vi "Reset Buffer Size.vi"(4 "Error In":errorcluster, 6 "Instance Name":T1, 7 "New Buffer Size":i32) -> (0 "Error Out":errorcluster)   [LabVIEW 2015, in "Temperature Controller Data Buffer.lvlib"]
uses:
  Temperature Controller Data Buffer.lvlib
  _libraries/Startup Processes/_typedefs/Subpanel Names.ctl
  _libraries/Startup Processes/Startup Processes.lvlib
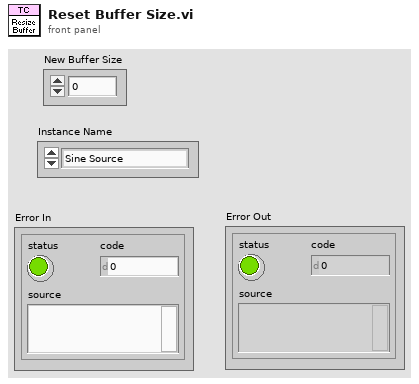
[diagram p1: front panel]
types:
  T1 = typedef "Startup Processes.lvlib/Subpanel Names.ctl" = enum16{"Sine Source", "Ramp Source", "Hen House TC", "Dog House TC", "Out House TC"}
  T2 = typedef "Temperature Controller Data Buffer.lvlib/buffer data typedef.ctl" = cluster{"TC Data":cluster{"Last value":dbl, "Error High Level":dbl, "Warning High Level":dbl, "Warning Low Level":dbl, "Error Low Level":dbl}[], "Counter":i32}
  T3 = cluster{"Last value":dbl, "Error High Level":dbl, "Warning High Level":dbl, "Warning Low Level":dbl, "Error Low Level":dbl}[]
  T4 = cluster{"Last value":dbl, "Error High Level":dbl, "Warning High Level":dbl, "Warning Low Level":dbl, "Error Low Level":dbl}
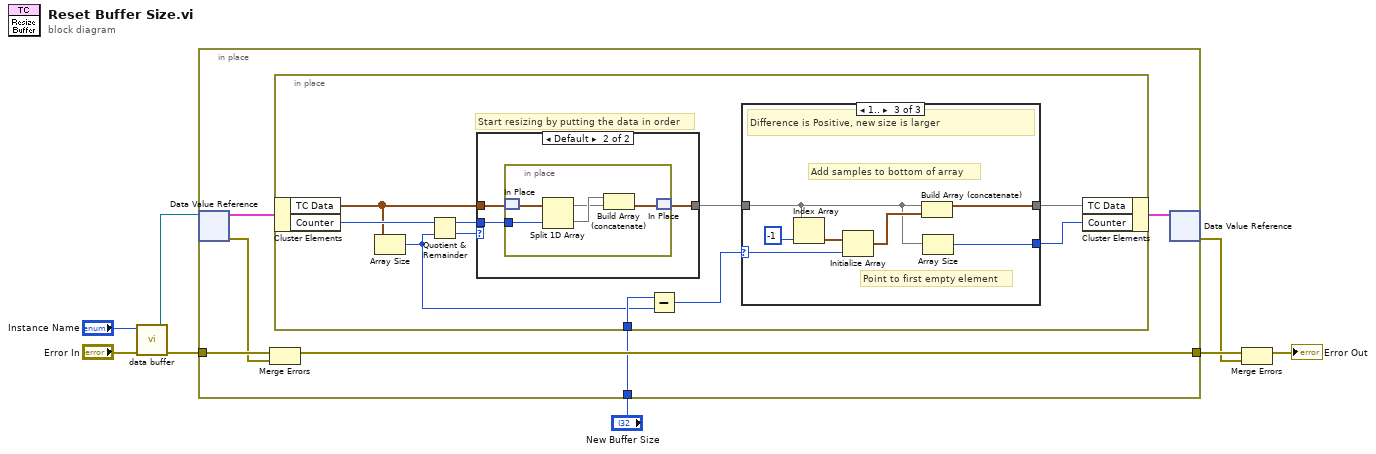
[diagram p0: block diagram]
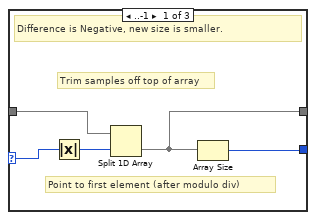
[diagram p2: hidden frame]
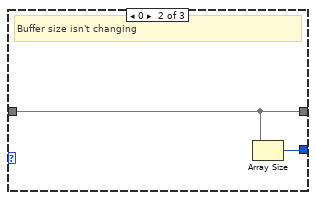
[diagram p3: hidden frame]
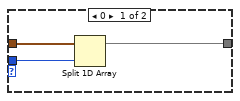
[diagram p4: hidden frame]
diagram:
  n1 = call "data buffer.vi"("Error In"="Error In", "Instance Name"="Instance Name") -> ("Error Out"=w6:errorcluster, "DVR"=w5:refnum<data-value>)  [unwired: 4 in]
  n2 = in-place {
    in-place-border: w6 -> [w14]
    in-place-border: [w13] -> w7
    in-place-border: "New Buffer Size" -> [w9]
    n3 = in-place-dvr #1(w5) -> (w11:T2, w12:errorcluster)
    n4 = Merge Errors(w14, w12) -> (w13:errorcluster)
    n5 = in-place {
      in-place-border: w9 -> [w16]
      # "Start resizing by putting the data in order"
      n6 = in-place-cluster #2(w11) -> ("TC Data"=w18:T3, "Counter"=w22:i32)
      n7 = Array Size(array=w18) -> (size(s)=w15:i32)
      n8 = Quotient & Remainder(x=w22, y=w15) -> (x-y*floor(x/y)=w23:i32, floor(x/y)=w24:i32)
      n9 = case shown="Default" w24 {
        tunnel: w18 -> [w41 w44]
        tunnel: [w39 w43] -> w21
        tunnel: w23 -> [w40 w42]
        frame 0 {
          n10 = Split 1D Array(array=w41, index=w40) -> (first subarray=w39:T3)  [unwired: 1 out]
        }
        frame Default {
          n11 = in-place {
            in-place-border: w42 -> [w49]
            n12 = in-place-match #3(w44) -> (w46:T3)
            n13 = Split 1D Array(array=w46, index=w49) -> (first subarray=w47:T3, second subarray=w48:T3)
            n14 = Build Array (concatenate)(w48, w47) -> (w45:T3)
            n15 = in-place-match #3(w45) -> (w43:T3)
          }
        }
      }
      n16 = Subtract(x=w16, y=w15) -> (x-y=w17:i32)
      n17 = case shown="1.." w17 {
        selector: w17 -> [w29 _ w38]
        tunnel: w21 -> [w27 w31 w33]
        tunnel: [w25 w30 w35] -> w20
        tunnel: [w26 w31 w36] -> w19
        frame ..-1 {
          # "Point to first element (after modulo div)"
          # "Trim samples off top of array"
          # "Difference is Negative, new size is smaller."
          n18 = Absolute Value(x=w29) -> (abs(x)=w28:i32)
          n19 = Split 1D Array(array=w27, index=w28) -> (second subarray=w26:T3)  [unwired: 1 out]
          n20 = Array Size(array=w26) -> (size(s)=w25:i32)
        }
        frame 0 {
          # "Buffer size isn't changing"
          n21 = Array Size(array=w31) -> (size(s)=w30:i32)
        }
        frame 1.. {
          # "Point to first empty element"
          # "Add samples to bottom of array"
          # "Difference is Positive, new size is larger"
          n22 = Index Array(array=w33, index=-1) -> (element=w34:T4)
          n23 = Initialize Array(w34, w38) -> (w37:T3)
          n24 = Build Array (concatenate)(w33, w37) -> (w36:T3)
          n25 = Array Size(array=w33) -> (size(s)=w35:i32)
        }
      }
      n26 = in-place-cluster #2("TC Data"=w19, "Counter"=w20) -> (w10:T2)
    }
    n27 = in-place-dvr #1(w10) -> (w4:errorcluster)  [unwired: 1 out]
  }
  n28 = Merge Errors(w7, w4) -> (→"Error Out":errorcluster)
